vi "Control Loop Process.vi"(8 "error in (no error)":errorcluster, 9 "MainDirectionIn":string, 11 "Main Process Class in":refnum<class "Main Class.lvclass">) -> (0 "error out":errorcluster, 1 "MainDirectionOut":string, 2 "ProcessAction":string[](array[string]), 3 "Main Process Class out":refnum<class "Main Class.lvclass">)   [LabVIEW 2019, in "Main Class.lvclass"]
uses:
  Main Class.lvclass
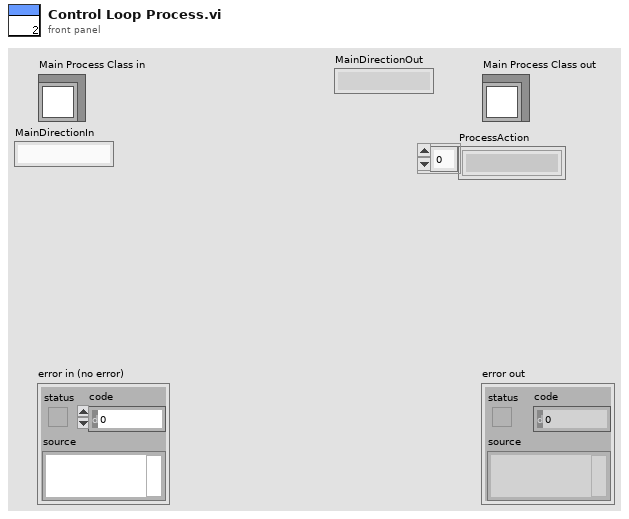
[diagram p1: front panel]
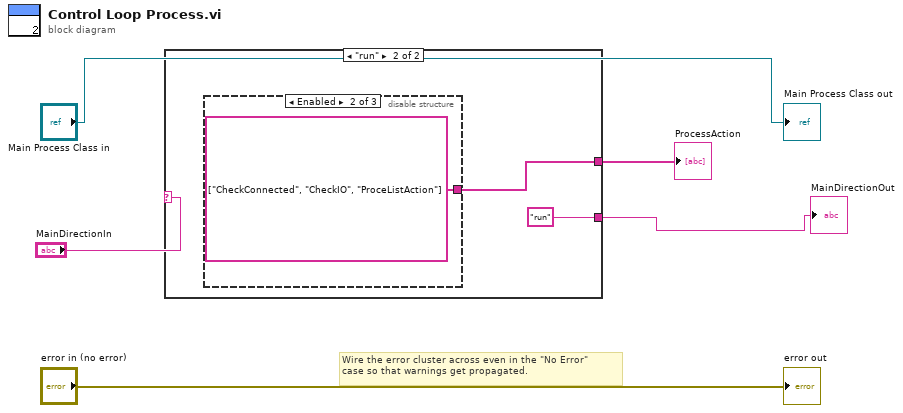
[diagram p0: block diagram]
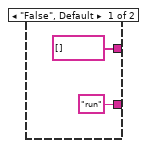
[diagram p2: hidden frame]
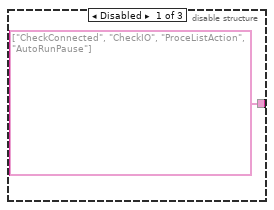
[diagram p3: hidden frame]
diagram:
  # "Wire the error cluster across even in the \"No Error\"\ncase so that warnings get propagated."
  n1 = case shown="\"run\"" "MainDirectionIn" {
    tunnel: ["run" "run"] -> w2
    tunnel: [string[] [] w8] -> w1
    frame "False", Default {
    }
    frame "run" {
      n2 = disable-structure shown="Enabled" {
        disable-tunnel: [string[] ["CheckConnected", "CheckIO", "ProceListAction", "AutoRunPause"] string[] ["CheckConnected", "CheckIO", "ProceListAction"] _] -> w8
        frame Disabled {
        }
        frame Enabled {
        }
        frame Disabled {
        }
      }
    }
  }
  "MainDirectionOut" <- w2
  "ProcessAction" <- w1
  "error out" <- "error in (no error)"
  "Main Process Class out" <- "Main Process Class in"
